vi "Exponent Function.vi"(1 "Exponent":dbl, 2 "In":dbl) -> (0 "Out":dbl)   [LabVIEW 2013]
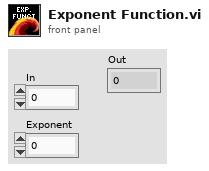
[diagram p1: front panel]
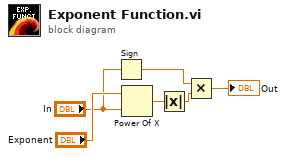
[diagram p0: block diagram]
diagram:
  n1 = Sign(1:"In") -> (0:w3:dbl)
  n2 = Power Of X(1:"In", 2:"Exponent") -> (0:w4:dbl)
  n3 = Absolute Value(x=w4) -> (abs(x)=w2:dbl)
  n4 = Multiply(x=w3, y=w2) -> (x*y=→"Out":dbl)
